vi "String Predicate.vi"(1 "Element":string) -> (0 "Value":bool)   [LabVIEW 2020, in "Tests.lvlib"]
uses:
  Tests.lvlib
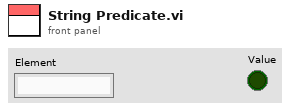
[diagram p1: front panel]
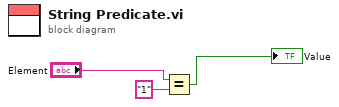
[diagram p0: block diagram]
diagram:
  n1 = Equal?(x="Element", y="1") -> (x = y?=→"Value":bool)
